vi "SampleHandler_move.vi"(8 "error in (no error)":errorcluster caption="エラー入力（エラーなし）", 10 "移動コマンド (G)":string="G,", 11 "VISAリソース名":refnum<visa-resource-name>) -> (0 "error out":errorcluster caption="エラー出力", 2 "停止状態":string, 3 "VISAリソース名出力":refnum<visa-resource-name>)   [LabVIEW 2017]
panel:
  out "文字列":string
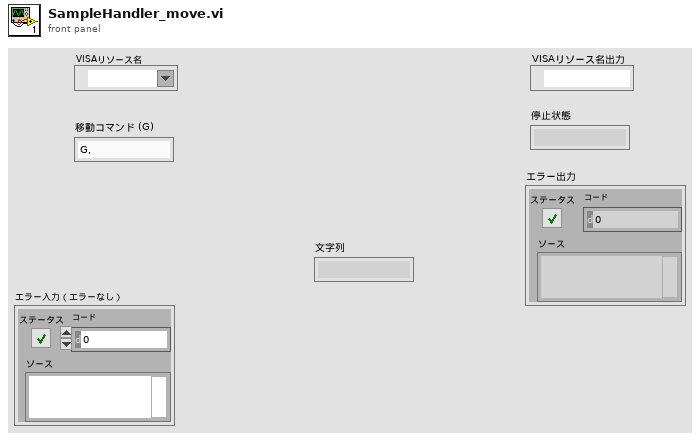
[diagram p1: front panel]
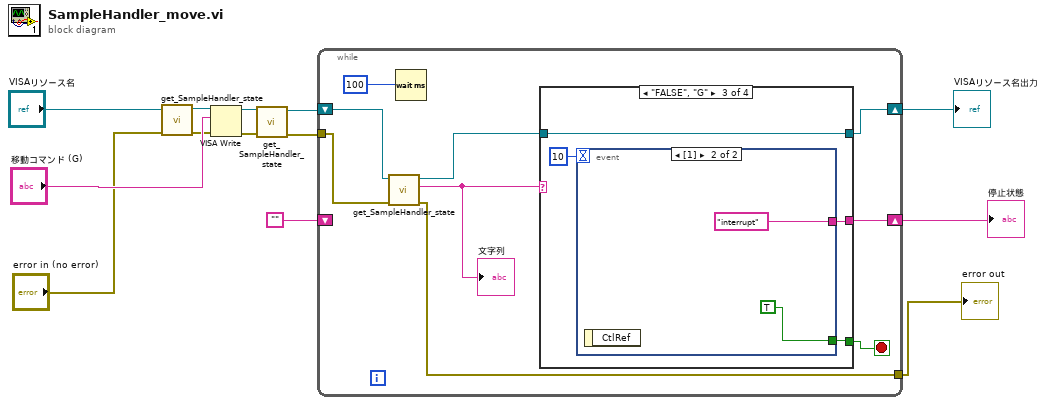
[diagram p0: block diagram]
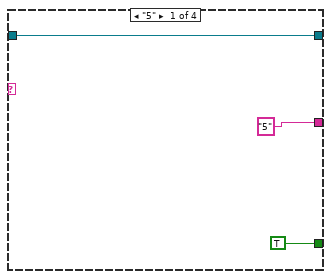
[diagram p2: hidden frame]
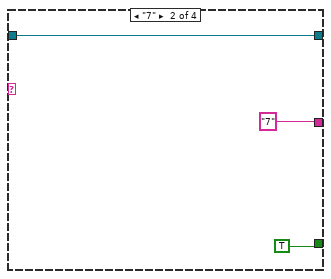
[diagram p3: hidden frame]
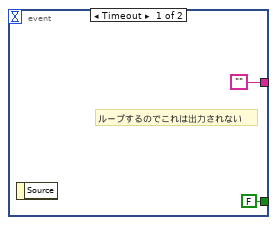
[diagram p4: hidden frame]
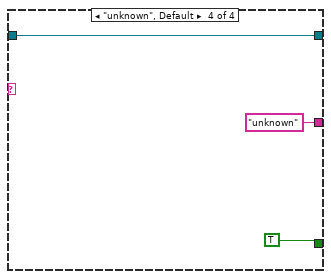
[diagram p5: hidden frame]
diagram:
  n1 = call "get_SampleHandler_state.vi"("error in (no error)"="error in (no error)", "VISAリソース名"="VISAリソース名") -> ("error out"=w7:errorcluster, "VISAリソース名（出力）"=w8:refnum<visa-resource-name>)  [unwired: 7 in, 1 out]
  n2 = VISA Write(VISA resource name=w8, write buffer="移動コマンド (G)", error in (no error)=w7) -> (VISA resource name out=w4:refnum<visa-resource-name>, error out=w2:errorcluster)  [unwired: 1 out]
  n3 = call "get_SampleHandler_state.vi"("error in (no error)"=w2, "VISAリソース名"=w4) -> ("error out"=w1:errorcluster, "VISAリソース名（出力）"=w3:refnum<visa-resource-name>)  [unwired: 7 in, 1 out]
  n4 = while {
    tunnel: w1 -> [w20]
    shift-right: [w18] -> w11
    shift-left: w3 -> [w21]
    tunnel: [w15] -> w10
    shift-right: [w16] -> w12
    shift-left: "" -> [_]
    stop <- w17 stop-if-true
    n5 = call "get_SampleHandler_state.vi"("error in (no error)"=w20, "VISAリソース名"=w21) -> ("error out"=w15:errorcluster, "response"=w14:string, "VISAリソース名（出力）"=w19:refnum<visa-resource-name>)  [unwired: 7 in]
    "文字列" <- w14
    n6 = Wait (ms)(milliseconds to wait=100) -> ()  [unwired: 1 out]
    n7 = case shown="\"FALSE\", \"G\"" w14 {
      tunnel: w19 -> [w25 w26 w32 w38]
      tunnel: [w25 w26 w32 w38] -> w18
      tunnel: [TRUE TRUE w31 TRUE] -> w17
      tunnel: ["5" "7" w30 "unknown"] -> w16
      frame "5" {
      }
      frame "7" {
      }
      frame "FALSE", "G" {
        n8 = event shown="[1]" {
          selector: _ -> [_ _]
          dyn-events: _ -> [_ _]
          timeout: 10 -> [_ _]
          tunnel: [FALSE TRUE] -> w31
          tunnel: ["" "interrupt"] -> w30
          event Timeout {
            # "ループするのでこれは出力されない"
            n9 = event-data() -> ()  [unwired: 1 in, 1 out]
          }
          event #1 (no event record) {
            n10 = event-data() -> ()  [unwired: 1 in, 1 out]
          }
        }
      }
      frame "unknown", Default {
      }
    }
  }
  "VISAリソース名出力" <- w11
  "停止状態" <- w12
  "error out" <- w10
